vi "simple_text.vi"() -> ()   [LabVIEW 2021]
panel:
  out "path":path
  out "text":string
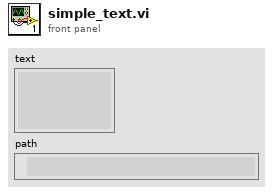
[diagram p1: front panel]
types:
  T1 = enum16{"open", "replace", "create", "open or create", "replace or create", "replace or create with confirmation"}
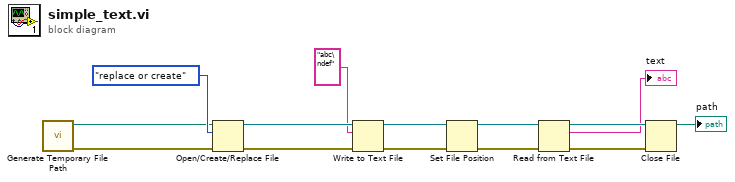
[diagram p0: block diagram]
diagram:
  n1 = call <vilib>:"Generate Temporary File Path.vi"() -> ("error out"=w13:errorcluster, "Unique Temporary File Path"=w12:path)  [unwired: 10 in]
  n2 = Open/Create/Replace File(file path (use dialog)=w12, error in=w13, operation (0:open)=T1."replace or create") -> (refnum out=w11:refnum<file>, error out=w9:errorcluster)  [unwired: 3 in, 1 out]
  n3 = Write to Text File(file (use dialog)=w11, text="abc\ndef", error in=w9) -> (refnum out=w10:refnum<file>, error out=w8:errorcluster)  [unwired: 1 in, 1 out]
  n4 = Set File Position(refnum=w10, error in=w8) -> (refnum out=w7:refnum<file>, error out=w6:errorcluster)  [unwired: 2 in]
  n5 = Read from Text File(file (use dialog)=w7, error in=w6) -> (refnum out=w4:refnum<file>, text=→"text":string, error out=w5:errorcluster)  [unwired: 2 in, 1 out]
  n6 = Close File(refnum=w4, error in=w5) -> (path=→"path":path)  [unwired: 1 out]
